vi "TestDouble.vi"(8 "error in":errorcluster, 11 "UnitTestFramework.lvclass in":refnum<class "UnitTestFramework.lvclass">) -> (0 "error out":errorcluster, 2 "Equal?":bool, 3 "UnitTestFramework.lvclass out":refnum<class "UnitTestFramework.lvclass">)   [LabVIEW 2019]
uses:
  UT/UnitTestFramework.lvclass
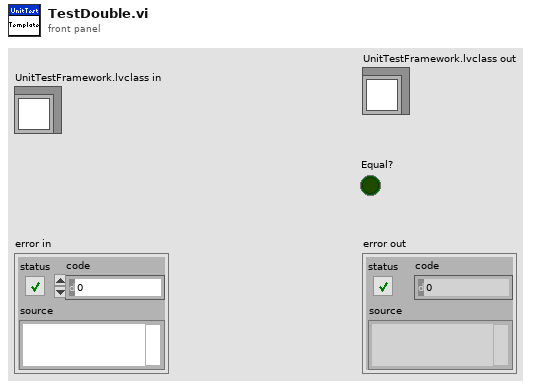
[diagram p1: front panel]
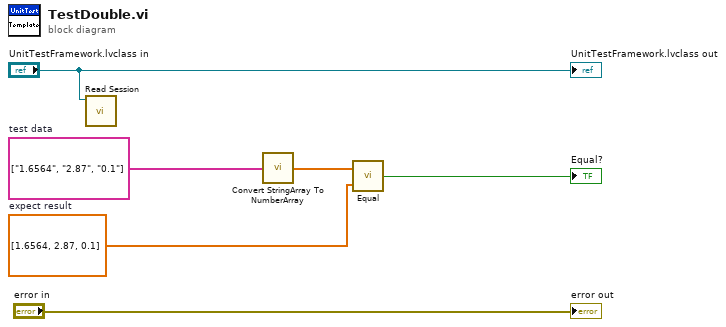
[diagram p0: block diagram]
diagram:
  w1 = dbl[] [1.6564, 2.87, 0.1]  # expect result
  w3 = string[] ["1.6564", "2.87", "0.1"]  # test data
  n1 = call-dynamic "Read Session.vi"("UnitTestFramework in"="UnitTestFramework.lvclass in") -> ()  [unwired: 8 in, 3 out]
  n2 = call "Convert StringArray To NumberArray.vi"("String Array"=w3) -> ("Nuber Array"=w2:dbl[])
  n3 = call "Equal.vi"("Y"=w1, "X"=w2) -> ("Equal?"=→"Equal?":bool)
  "UnitTestFramework.lvclass out" <- "UnitTestFramework.lvclass in"
  "error out" <- "error in"
